vi "Magnet manager.vi"(8 "Queue to UI":T1, 11 "Module queue":T1) -> ()   [LabVIEW 2021, in "Magnet module.lvlib"]
doc: "Magnet module controls: power supply unit (PSU/SMS) and temperature monitor (TM/LSC218).\nPSU controls mainly: switch heater and ramping of current which runs throught coil.\nTM controls temperature of switch, coil and cryostat.\nMessage for magnet is a cluster that contains: {(enum) Command , (variant) Data}\nFor simplifieing of documentation, the Command is noted as a name of instruction, and Data is represented by a requered datatype (mostly cluster) name.\nCommands:\nInitialize(Magnet Config Constants) - Sugesstion: Load configuration constants from configuration file.\nSet field (Set field{B, R, cr}) - B-field[T], R-ramp[A/s], cr - custom ramp[bool].\nSwitch mode(mode) - to persistant, or to ramping.\nBlackout() - undone functionality of emergency deenergizing.\nUpdate() - Important! This triggers update of data from instruments. Shoud occure in regular intervals as priority message.\nResponses:\nMagnet initialized ();\nTM revision(temperature monitor revision);\nMagnet init error(error);\nSetting field(Set Field{B, R, cr});\nWarning(string);\nSwitching to(mode);\nUpdate error(error);\nTM update(TM sensors);\nPSU update(PSU data);\nMagnet status();"
uses:
  Magnet module.lvlib
  ctl/Magnet Orders.ctl
  ctl/MSG to magnet.ctl
  ctl/Magnet module states.ctl
  Messenger service/MessengerLib.lvlib
  Messenger service/Data types/Mailbox address.ctl
panel:
  out "Ended":bool=TRUE
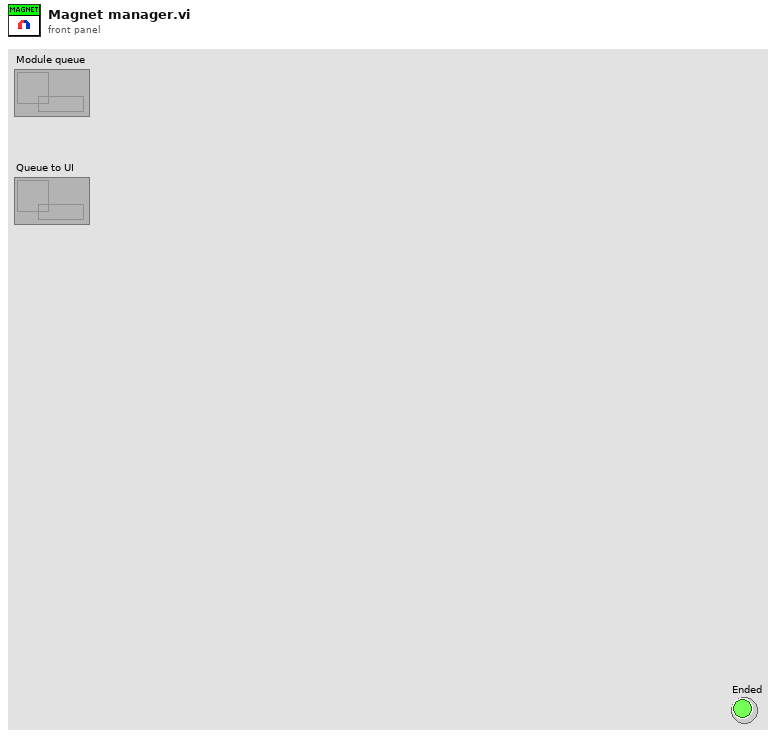
[diagram p1: front panel]
types:
  T1 = typedef "MessengerLib.lvlib/Mailbox address.ctl" = refnum<queue>
  T2 = typedef "Magnet module states.ctl" = enum16{"Initialize", "Connect to TM", "Connect to PSU", "Get update from TM", "Get update from PSU", "Set PSU", "Disconnect TM", "Disconnect PSU", "End"}
  T3 = typedef "Magnet module.lvlib/MSG to magnet.ctl" = cluster{"Order":T4, "Data":variant}
  T4 = typedef "Magnet module.lvlib/Magnet Orders.ctl" = enum16{"Ignore", "Connect", "Update", "Switch mode", "Set field", "Stop ramping", "Equalize output", "Zero output", "Flip polarity", "Blackout", "Set timer", "Eval temperatures", "Disconnect"}
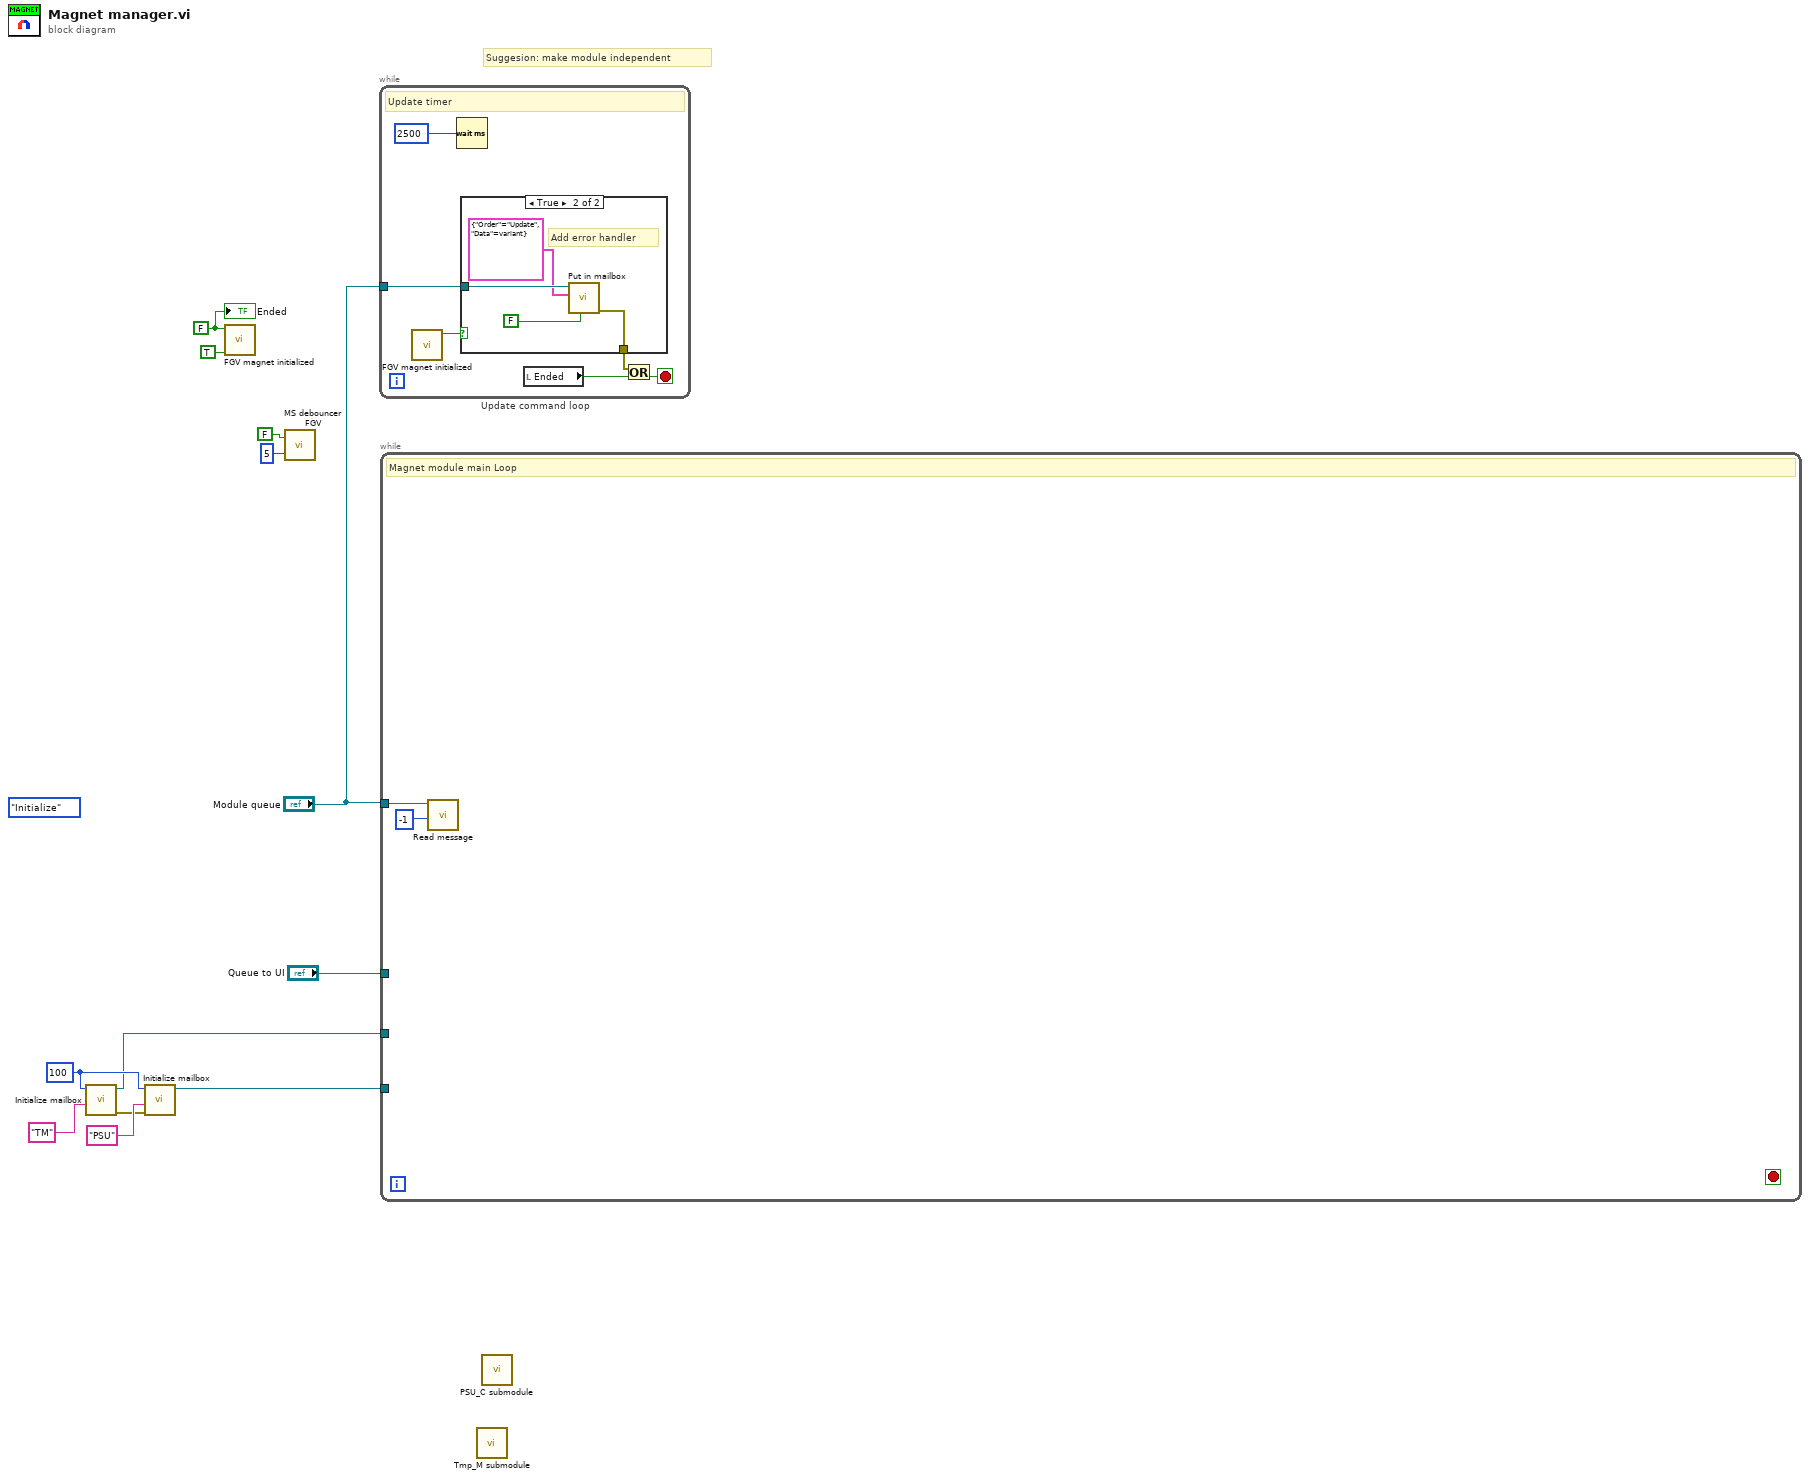
[diagram p0: block diagram]
diagram:
  w4 = 100 ("MailboxSize(-1)")
  (unwired) Magnet_module_states."Initialize"
  w8 = FALSE ("Initialized in")
  # "Suggesion: make module independent"
  n1 = call "Initialize mailbox.vi"("name (unnamed)"="TM", "MailboxSize(-1)"=w4) -> ("error out"=w5:errorcluster, "Queue out"=w2:refnum<queue>)  [unwired: 8 in]
  n2 = call "Initialize mailbox.vi"("error in"=w5, "name (unnamed)"="PSU", "MailboxSize(-1)"=w4) -> ("Queue out"=w1:refnum<queue>)  [unwired: 7 in, 1 out]
  n3 = call "FGV magnet initialized.vi"("Write?(F)"=TRUE, "Initialized in"=w8) -> ()  [unwired: 9 in, 1 out]
  n4 = call "MS debouncer FGV.vi"("Iterations"=5, "At target?"=FALSE ("On target?")) -> ()  [unwired: 1 out]
  n5 = while "Update command loop" {
    tunnel: "Module queue" -> [w17]
    stop <- w14 stop-if-true
    # "Update timer"
    n6 = call "FGV magnet initialized.vi"() -> ("Initialized out"=w16:bool)  [unwired: 11 in]
    n7 = Wait (ms)(milliseconds to wait=u32 2500) -> ()  [unwired: 1 out]
    n8 = case shown="True" w16 {
      tunnel: w17 -> [_ w22]
      tunnel: [_ w19] -> w13
      frame False {
      }
      frame True {
        # "Add error handler"
        n9 = call "Put in mailbox.vi"("Priority? (F)"=FALSE ("Priority?"), "Message"=T3 {"Order"=enum."Update", "Data"=variant(enum16{"Ramping", "Perzistant"} enum."Ramping")} ("MSG to magnet"), "Queue in"=w22) -> ("error out"=w19:errorcluster)  [unwired: 6 in, 2 out]
      }
    }
    n10 = local read "Ended"() -> (w15:bool)
    n11 = Or(x=w13, y=w15) -> (x .or. y?=w14:bool)
  }
  n12 = while {
    tunnel: "Module queue" -> [w24]
    tunnel: "Queue to UI" -> [_]
    tunnel: w2 -> [_]
    tunnel: w1 -> [_]
    stop <- _ stop-if-true
    # "Magnet module main Loop"
    n13 = call "Read message.vi"("timeout in ms (10)"=-1 ("timeout in ms (-1)"), "Module queue ref"=w24) -> ()  [unwired: 8 in, 2 out]
  }
  n14 = call "Tmp_M submodule.vi"() -> ()  [unwired: 10 in, 2 out]
  n15 = call "PSU_C submodule.vi"() -> ()  [unwired: 12 in]
  "Ended" <- w8
